vi "tankcontrol.vi"(1 "dt":dbl, 2 "h(n)":dbl, 3 "Fout [cm3/s]":dbl, 4 "U [V]":dbl) -> (0 "h(n+1)":dbl)   [LabVIEW 2021]
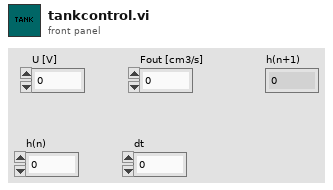
[diagram p1: front panel]
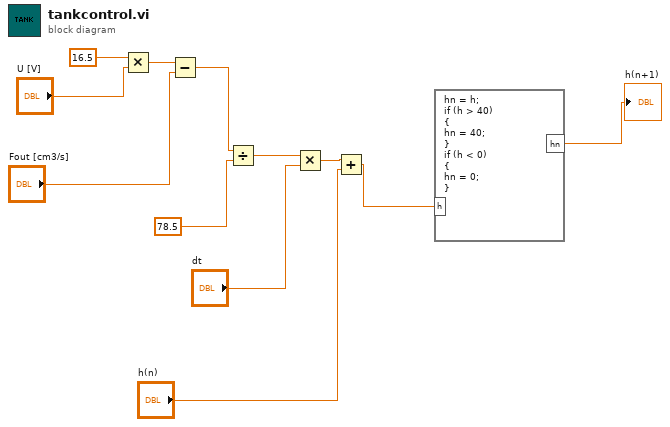
[diagram p0: block diagram]
diagram:
  n1 = Multiply(x=16.5, y="U [V]") -> (x*y=w10:dbl)
  n2 = Subtract(x=w10, y="Fout [cm3/s]") -> (x-y=w12:dbl)
  n3 = Divide(x=w12, y=78.5) -> (x/y=w6:dbl)
  n4 = Multiply(x=w6, y="dt") -> (x*y=w4:dbl)
  n5 = Add(x=w4, y="h(n)") -> (x+y=w2:dbl)
  n6 = formula code="hn = h;\nif (h > 40)\n{\nhn = 40;\n}\nif (h < 0)\n{\nhn = 0;\n}"("h"=w2) -> ("hn"=→"h(n+1)":dbl)
